vi "Convert View 3x3 to Arrays.vi"(0 "I32 3x3 Grid":T2) -> (2 "Directions Out":T1[](array[typedef]), 3 "Values Out":i32[](array[numeric]))   [LabVIEW 2016, in "AntFarm_MB.lvclass"]
uses:
  AntFarm_MB.lvclass
  TypeDefs/Cluster_I32 3x3 Grid.ctl
  Type Defs/Direction Enum.ctl
  Type Defs/SB Type Defs.lvlib
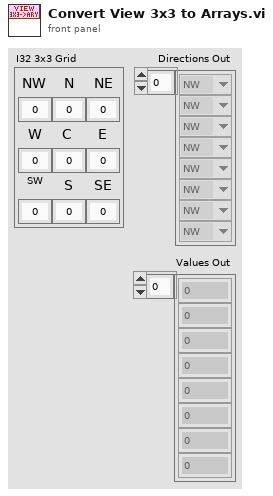
[diagram p1: front panel]
types:
  T1 = typedef "SB Type Defs.lvlib/Direction Enum.ctl" = enum16{"NW", "N", "NE", "E", "SE", "S", "SW", "W"}
  T2 = typedef "Cluster_I32 3x3 Grid.ctl" = cluster{"NW":i32, "N":i32, "NE":i32, "E":i32, "SE":i32, "S":i32, "SW":i32, "W":i32, "C":i32}
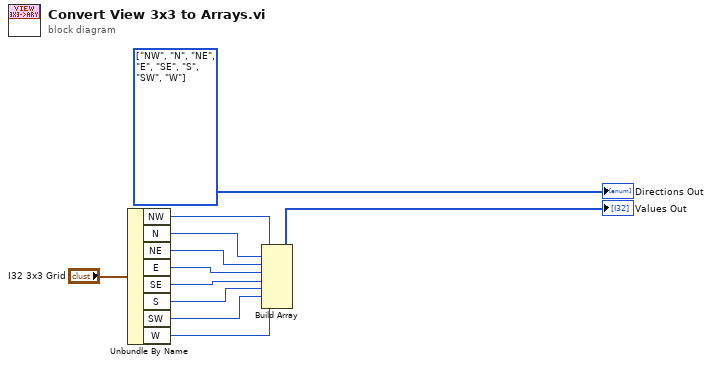
[diagram p0: block diagram]
diagram:
  w10 = T1[] [enum."NW", enum."N", enum."NE", enum."E", enum."SE", enum."S", enum."SW", enum."W"] items=["NW", "N", "NE", "E", "SE", "S", "SW", "W"] ("Directions Out")
  n1 = Unbundle By Name("I32 3x3 Grid") -> ("NW"=w9:i32, "N"=w6:i32, "NE"=w4:i32, "E"=w2:i32, "SE"=w3:i32, "S"=w5:i32, "SW"=w7:i32, "W"=w8:i32)
  n2 = Build Array(w9, w6, w4, w2, w3, w5, w7, w8) -> (→"Values Out":i32[])
  "Directions Out" <- w10
